vi "runPushing.vi"(4 "Service? in":bool, 5 "Distance":dbl, 6 "Fault?":bool, 7 "Time":dbl, 8 "error in (no error)":errorcluster, 9 "Actuators in":T1, 10 "State in":T2, 11 "FullRun in":refnum<class "FullRun.lvclass">) -> (0 "error out":errorcluster, 1 "Actuators out":T1, 2 "State out":T2, 3 "FullRun out":refnum<class "FullRun.lvclass">)   [LabVIEW 2017, in "ControlLibrary.lvlib" / "FullRun.lvclass"]
uses:
  FullRun.lvclass
  TypeDef_ControlState.ctl
  TypeDef_DigitalOuts.ctl
  RunTypeClass/RunType.lvclass
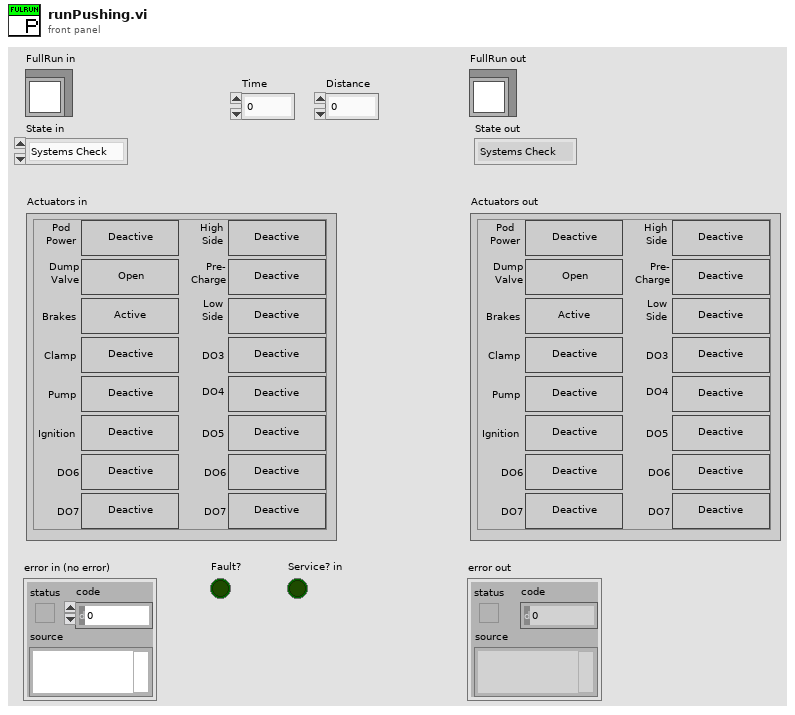
[diagram p1: front panel]
types:
  T1 = typedef "TypeDef_DigitalOuts.ctl" = cluster{"Pod Power":bool, "Dump Valve":bool, "Brakes":bool, "Clamp":bool, "Pump":bool, "Ignition":bool, "DO6":bool, "DO7":bool, "HighSide":bool, "Precharge":bool, "LowSide":bool, "DO3":bool, "DO4":bool, "DO5":bool, "DO62":bool, "DO72":bool}
  T2 = typedef "TypeDef_ControlState.ctl" = enum16{"Systems Check", "Idle", "Ready", "Pushing", "Coast", "Braking", "Fault", "Shutdown", "Service", "Precharge", "Blank"}
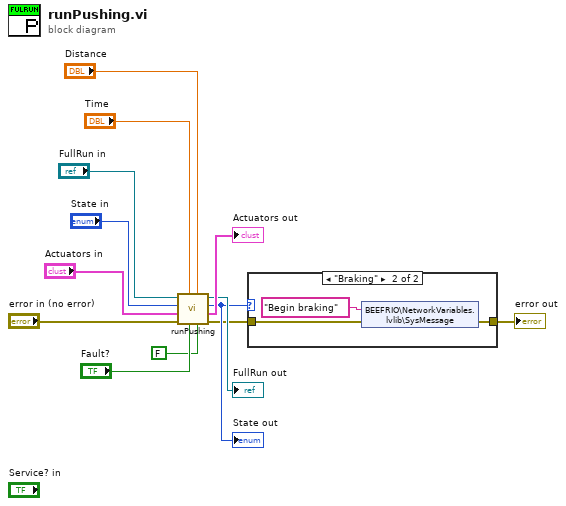
[diagram p0: block diagram]
diagram:
  n1 = call-parent "runPushing.vi"("Service? in"=FALSE, "Distance"="Distance", "Fault?"="Fault?", "Time"="Time", "error in (no error)"="error in (no error)", "Actuators in"="Actuators in", "State in"="State in", "RunType in"="FullRun in") -> ("error out"=w2:errorcluster, "Actuators out"=→"Actuators out":T1, "State out"=w3:T2, "RunType out"=→"FullRun out":refnum<class "FullRun.lvclass">)
  "State out" <- w3
  n2 = case shown="\"Braking\"" w3 {
    tunnel: w2 -> [w14 w16]
    tunnel: [w14 w15] -> w1
    frame Default {
    }
    frame "Braking" {
      n3 = shared-variable "BEEFRIO\\NetworkVariables.lvlib\\SysMessage"("Begin braking" ("SysMessage"), error in=w16) -> (error out=w15:errorcluster)
    }
  }
  "error out" <- w1
